vi "EnQ Sample.vi"(8 "error in (no error)":errorcluster, 10 "Sample.lvclass":refnum<class "Sample.lvclass">, 11 "Transfer Line in":refnum<class "Transfer Line.lvclass">) -> (0 "error out":errorcluster, 3 "Transfer Line out":refnum<class "Transfer Line.lvclass">)   [LabVIEW 2015, in "cRIO-Carbondioxide.lvlib" / "CO2-Actor.lvlib" / "Transfer Line.lvclass"]
uses:
  Transfer Line.lvclass
  subs/Sample/Sample.lvclass
  Transfer Line.lvclass/Transfer Line.ctl
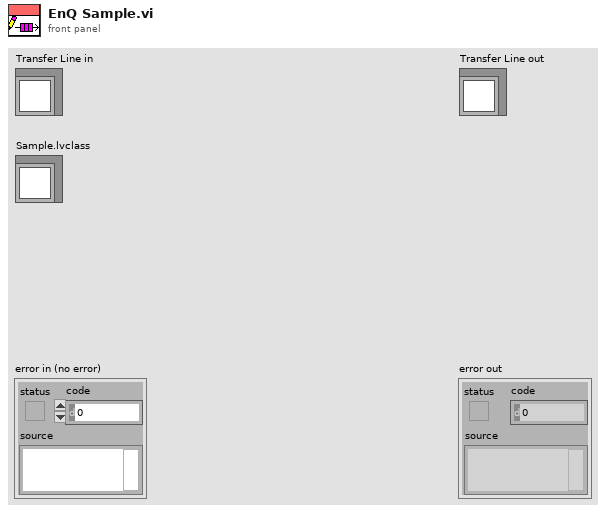
[diagram p1: front panel]
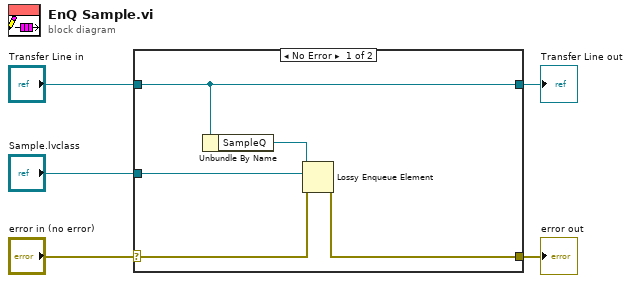
[diagram p0: block diagram]
diagram:
  n1 = case shown="No Error" "error in (no error)" {
    selector: "error in (no error)" -> [w8 w11]
    tunnel: [w7 w11] -> w4
    tunnel: [w10 w12] -> w2
    tunnel: "Transfer Line in" -> [w10 w12]
    tunnel: "Sample.lvclass" -> [w6 _]
    frame No Error {
      n2 = Unbundle By Name(w10) -> ("SampleQ"=w9:refnum<queue>)
      n3 = Lossy Enqueue Element(queue=w9, element=w6, error in (no error)=w8) -> (error out=w7:errorcluster)  [unwired: 3 out]
    }
    frame Error {
    }
  }
  "error out" <- w4
  "Transfer Line out" <- w2
